vi "Read Com Port.vi"(8 "error in (no error)":errorcluster, 11 "SpinCoater in":refnum<class "SpinCoater.lvclass">) -> (0 "error out":errorcluster, 2 "Com Port":refnum<visa-resource-name>, 3 "SpinCoater out":refnum<class "SpinCoater.lvclass">)   [LabVIEW 2020, in "SpinCoater.lvclass"]
uses:
  <instrlib>/Classes/SpinCoater/SpinCoater.lvclass
  <instrlib>/Classes/SpinCoater/SpinCoater.lvclass/SpinCoater.ctl
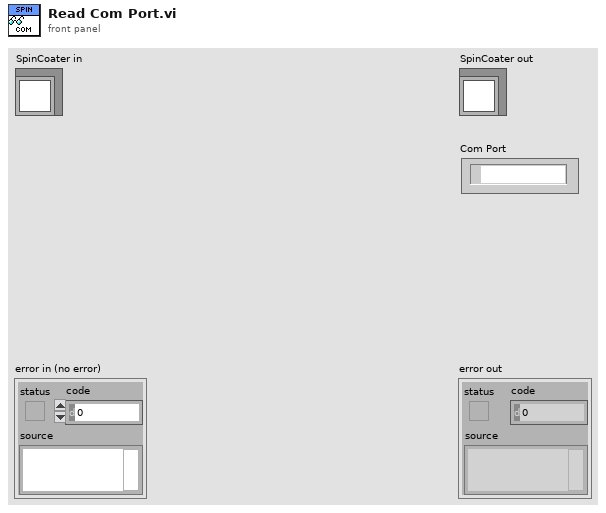
[diagram p1: front panel]
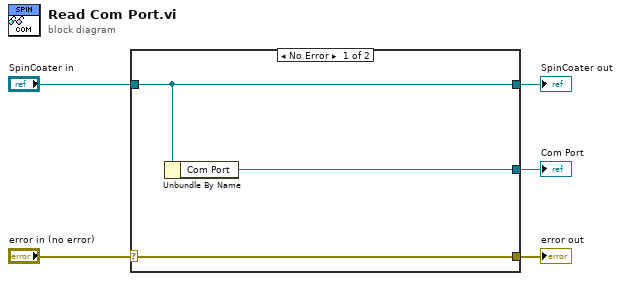
[diagram p0: block diagram]
diagram:
  n1 = case shown="No Error" "error in (no error)" {
    selector: "error in (no error)" -> [w8 w9]
    tunnel: [w8 w9] -> w4
    tunnel: [w7 w10] -> w2
    tunnel: "SpinCoater in" -> [w7 w10]
    tunnel: [w6 _] -> w1
    frame No Error {
      n2 = Unbundle By Name(w7) -> ("Com Port"=w6:refnum<visa-resource-name>)
    }
    frame Error {
    }
  }
  "error out" <- w4
  "SpinCoater out" <- w2
  "Com Port" <- w1
